vi "Get Current Data Str By ID V.vi"(8 "error in (no error)":errorcluster, 9 "bufferLength":i16, 10 "s":string, 11 "id":u32) -> (0 "error out":errorcluster, 2 "s out":string, 3 "function return":i16)   [LabVIEW 2009, in "VantagePro.lvlib"]
doc: "DllAccess short int _stdcall GetCurrentDataStrByID_V (DWORD id, char *s, short int bufferLength);"
uses:
  VantagePro.lvlib
  <userlib>/VantagePro/VantagePro.dll
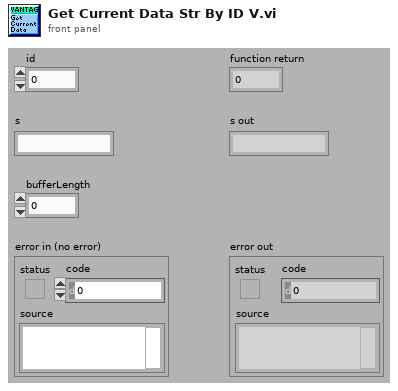
[diagram p1: front panel]
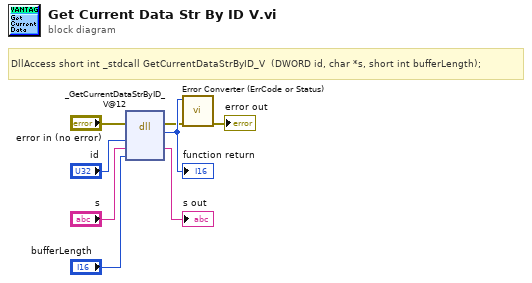
[diagram p0: block diagram]
diagram:
  # "DllAccess short int _stdcall GetCurrentDataStrByID_V  (DWORD id, char *s, short int bufferLength);"
  n1 = dll-call lib="C:/Program Files/National Instruments/LabVIEW 2010/user.lib/VantagePro/VantagePro.*" fn="_GetCurrentDataStrByID_V@12"(error in="error in (no error)", "id"="id", "s"="s", "bufferLength"="bufferLength") -> (error out=w2:errorcluster, w8:i16, "s"=→"s out":string)  [unwired: 4 in, 1 out]
  "function return" <- w8
  n2 = call "Error Converter (ErrCode or Status).vi"("error in (no error)"=w2, "error code"=w8) -> ("error out"=→"error out":errorcluster)  [unwired: 9 in]
